vi "ChooseDirection.vi"(6 "Boolean":bool, 8 "y in":i32, 9 "x in":i32, 11 "Start Goal Data":T1) -> (0 "y out":i32, 1 "x out 2":i32, 3 "Start Goal Data out":T1)   [LabVIEW 2013]
uses:
  Bug_StartGoalData.ctl
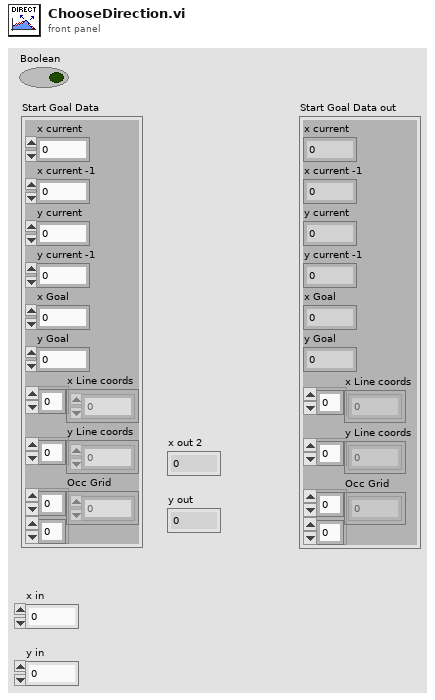
[diagram p1: front panel]
types:
  T1 = typedef "Bug_StartGoalData.ctl" = cluster{"x current":i32, "x current -1":i32, "y current":i32, "y current -1":i32, "x Goal":i32, "y Goal":i32, "x Line coords":i32[], "y Line coords":i32[], "Occ Grid":dbl[][]}
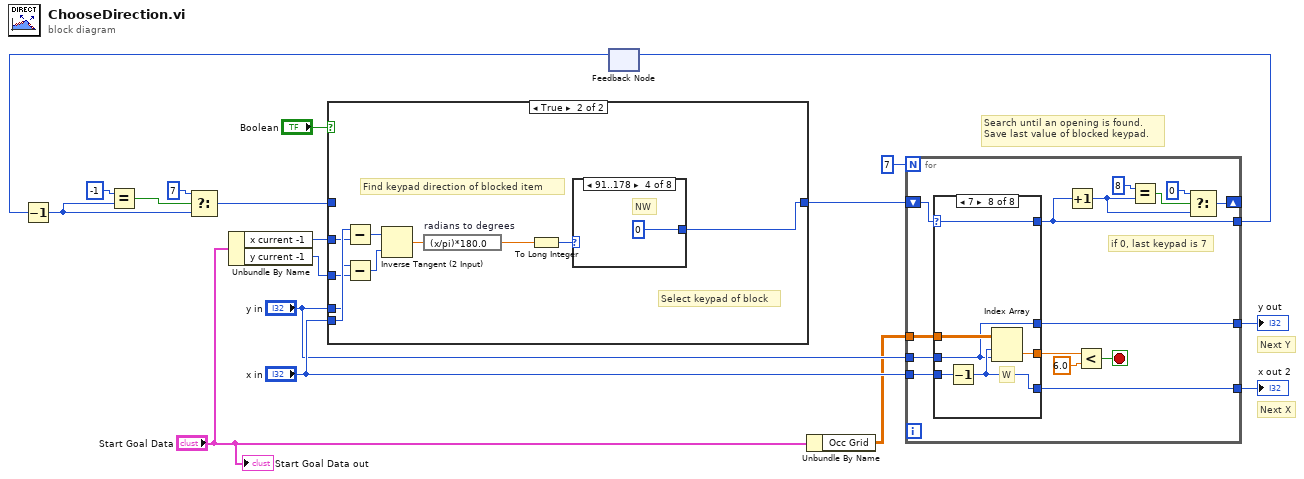
[diagram p0: block diagram]
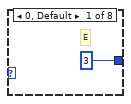
[diagram p3: hidden frame]
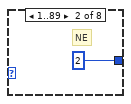
[diagram p4: hidden frame]
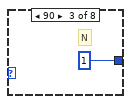
[diagram p5: hidden frame]
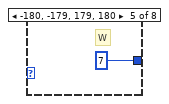
[diagram p6: hidden frame]
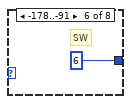
[diagram p7: hidden frame]
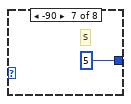
[diagram p8: hidden frame]
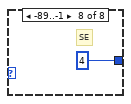
[diagram p9: hidden frame]
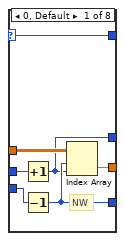
[diagram p10: hidden frame]
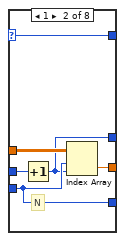
[diagram p11: hidden frame]
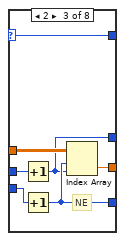
[diagram p12: hidden frame]
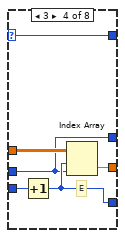
[diagram p13: hidden frame]
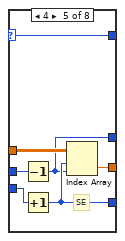
[diagram p14: hidden frame]
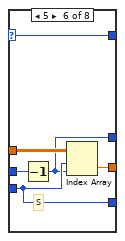
[diagram p15: hidden frame]
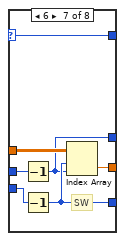
[diagram p16: hidden frame]
diagram:
  # "Search until an opening is found.\nSave last value of blocked keypad."
  # "Next Y"
  # "Next X"
  n1 = Unbundle By Name("Start Goal Data") -> ("x current -1"=w17:i32, "y current -1"=w18:i32)
  n2 = feedback #1() -> (w9:i32)  [unwired: 1 in]
  n3 = Decrement(x=w9) -> (x-1=w13:i32)
  n4 = Equal?(x=-1, y=w13) -> (x = y?=w11:bool)
  n5 = Select(t=7, s=w11, f=w13) -> (s? t:f=w14:i32)
  n6 = case shown="True" "Boolean" {
    tunnel: w17 -> [_ w22]
    tunnel: "x in" -> [_ w23]
    tunnel: [w19 w27] -> w7
    tunnel: w18 -> [_ w20]
    tunnel: "y in" -> [_ w21]
    tunnel: w14 -> [w19 _]
    frame False {
    }
    frame True {
      # "Select keypad of block"
      # "Find keypad direction of blocked item"
      n7 = Subtract(x=w23, y=w22) -> (x-y=w28:i32)
      n8 = Subtract(x=w21, y=w20) -> (x-y=w29:i32)
      n9 = Inverse Tangent (2 Input)(1:w29, 2:w28) -> (0:w26:dbl)
      n10 = expression code="(x/pi)*180.0" "radians to degrees"(w26) -> (w25:dbl)
      n11 = To Long Integer(number=w25) -> (32bit integer=w24:i32)
      n12 = case shown="91..178" w24 {
        tunnel: [3 2 1 0 7 6 5 4] -> w27
        frame 0, Default {
          # "E"
        }
        frame 1..89 {
          # "NE"
        }
        frame 90 {
          # "N"
        }
        frame 91..178 {
          # "NW"
        }
        frame -180, -179, 179, 180 {
          # "W"
        }
        frame -178..-91 {
          # "SW"
        }
        frame -90 {
          # "S"
        }
        frame -89..-1 {
          # "SE"
        }
      }
    }
  }
  n13 = Unbundle By Name("Start Goal Data") -> ("Occ Grid"=w1:dbl[][])
  n14 = for {
    N: 7 -> [_]
    tunnel: w1 -> [w51]
    shift-right: [w43] -> _
    shift-left: w7 -> [w52]
    tunnel: "x in" -> [w50]
    tunnel: "y in" -> [w49]
    tunnel: [w45] -> w5
    tunnel: [w44] -> w6
    tunnel: [w38] -> w16
    stop <- w46 stop-if-true
    # "if 0, last keypad is 7"
    n15 = case shown="7" w52 {
      selector: w52 -> [w59 w65 w72 w78 w85 w91 w98 w104]
      tunnel: w51 -> [w58 w64 w71 w77 w84 w90 w97 w103]
      tunnel: [w59 w65 w72 w78 w85 w91 w98 w104] -> w38
      tunnel: w50 -> [w57 w61 w69 w75 w83 w87 w96 w102]
      tunnel: w49 -> [w56 w62 w67 w73 w82 w89 w95 w99]
      tunnel: [w55 w63 w70 w76 w81 w88 w94 w101] -> w48
      tunnel: [w54 w61 w68 w74 w80 w87 w93 w100] -> w45
      tunnel: [w53 w60 w66 w73 w79 w86 w92 w99] -> w44
      frame 0, Default {
        # "NW"
        n16 = Increment(x=w56) -> (x+1=w53:i32)
        n17 = Decrement(x=w57) -> (x-1=w54:i32)
        n18 = Index Array(array=w58, index (row)=w54, index (col)=w53) -> (element=w55:dbl)
      }
      frame 1 {
        # "N"
        n19 = Increment(x=w62) -> (x+1=w60:i32)
        n20 = Index Array(array=w64, index (row)=w61, index (col)=w60) -> (element=w63:dbl)
      }
      frame 2 {
        # "NE"
        n21 = Increment(x=w67) -> (x+1=w66:i32)
        n22 = Increment(x=w69) -> (x+1=w68:i32)
        n23 = Index Array(array=w71, index (row)=w68, index (col)=w66) -> (element=w70:dbl)
      }
      frame 3 {
        # "E"
        n24 = Increment(x=w75) -> (x+1=w74:i32)
        n25 = Index Array(array=w77, index (row)=w74, index (col)=w73) -> (element=w76:dbl)
      }
      frame 4 {
        # "SE"
        n26 = Decrement(x=w82) -> (x-1=w79:i32)
        n27 = Increment(x=w83) -> (x+1=w80:i32)
        n28 = Index Array(array=w84, index (row)=w80, index (col)=w79) -> (element=w81:dbl)
      }
      frame 5 {
        # "S"
        n29 = Decrement(x=w89) -> (x-1=w86:i32)
        n30 = Index Array(array=w90, index (row)=w87, index (col)=w86) -> (element=w88:dbl)
      }
      frame 6 {
        # "SW"
        n31 = Decrement(x=w95) -> (x-1=w92:i32)
        n32 = Decrement(x=w96) -> (x-1=w93:i32)
        n33 = Index Array(array=w97, index (row)=w93, index (col)=w92) -> (element=w94:dbl)
      }
      frame 7 {
        # "W"
        n34 = Decrement(x=w102) -> (x-1=w100:i32)
        n35 = Index Array(array=w103, index (row)=w100, index (col)=w99) -> (element=w101:dbl)
      }
    }
    n36 = Increment(x=w38) -> (x+1=w41:i32)
    n37 = Less?(x=w48, y=6.0) -> (x < y?=w46:bool)
    n38 = Equal?(x=8, y=w41) -> (x = y?=w42:bool)
    n39 = Select(t=0, s=w42, f=w41) -> (s? t:f=w43:i32)
  }
  "y out" <- w6
  "x out 2" <- w5
  n40 = feedback-in #1(w16) -> ()
  "Start Goal Data out" <- "Start Goal Data"
